vi "ReadData.vi"() -> (7 "Data":T1={"DAQ Config Data"={"Vertical"={"Coupling"=1, "Offset (V)"=-0.5, "Range (V)"=2.0, "Impedance"=50.0}, "Horizontal"={"Offset Time"=0.0, "Sample Time (S)"=22.0, "Sample Points"=1000}, "Trigger\n"={"Lower Level (V)"=-0.02, "Trigger Slope"=1, "Trigger Source"=10}, "Acquisition"={"Trigger Mode"=1, "Initiate Continuously"=0, "Acquire Type"=0, "Acquire Count"=1}, "Channel"=0, "Instrument Handle"=0, "Error"={"status"=FALSE, "code"=0, "source"=""}, "State"=1}, "Acquisition"={"Current"={"Acquiring Now?"=FALSE, "Waveforms Acquired"=0.0, "Start of Acquisition"=timestamp(0 s since 1904-01-01), "Acquisition Name"=""}, "Stop Condition"={"Quota"=3000.0, "Duration (S)"=22, "Stop Condition"=FALSE}, "Config Needed"=FALSE}, "Measurement"={"Waveform"={"t0"=timestamp(0 s since 1904-01-01), "dt"=1.0, "Y"=[]}, "Peak Heights"=[], "Acquisition Time"=timestamp(0 s since 1904-01-01), "File Path"=path "C:/Users/lab-341/Desktop/Reed/Oscilloscope VI/pulses.tdms", "TDMS File Handle"=refnum}, "UI References"={"Acquire"=refnum, "Configure DAQ"=refnum, "Measurement (Ch1)"=refnum, "Update Needed?"=FALSE, "New Run"=refnum, "Signal"=refnum}, "Run Info"={"Active Run?"=FALSE, "Run Notes"="Enter in notes explaining the purpose of the run and any unusual steps taken in the process. This should make it clear why the data was taken. e.g. \"Measuring LXe scintillation light with Teflon\" or \"Measuring dark pulses to determine SPE gain.\" Concise is good but precise is better.", "User Name"="", "Campaign ID#"="", "Run Name"="", "Start Time"=timestamp(0 s since 1904-01-01), "End Time"=timestamp(0 s since 1904-01-01)}, "System Status"={"Bias Voltage"=0.0, "SiPM Temperature"=[], "Slow Control User"="", "LXe"=0.0}, "Acquisition Info"={"Trigger Mode"=FALSE, "Acquisition Mode"=FALSE, "Bias Voltage (V)"=0.0, "Preamplifier"=0, "Shaping Amplifier"=0, "Acquisition Notes"="", "1"=FALSE, "2"=FALSE}} {"Acquisition Info"."Shaping Amplifier" items=["CR-200-100ns", "CR-200-1us"]; "Acquisition Info"."Preamplifier" items=["CR-Z-113-1k", "CR-Z-113-5k", "CR-Z-SiPM"]; "DAQ Config Data"."State" items=["Enable"=1, "Disable"=0]; "DAQ Config Data"."Channel" items=["Input Channel 1", "Input Channel 2", "Input Channel 3", "Input Channel 4"]; "DAQ Config Data"."Acquisition"."Acquire Type" items=["Normal"=0, "Average"=1, "Envelope"=2, "Peak Detect"=3, "High Resolution"=4, "Fast"=5, "Equivalent Time"=16]; "DAQ Config Data"."Acquisition"."Initiate Continuously" items=["Continuously"=1, "Single Capture"=0]; "DAQ Config Data"."Acquisition"."Trigger Mode" items=["Auto", "Normal"]; "DAQ Config Data"."Trigger"."Trigger Source" items=["TTL0", "TTL1", "TTL2", "TTL3", "TTL4", "TTL5", "TTL6", "TTL7", "ECL0", "ECL1", "Input Channel 1", "Input Channel 2", "Input Channel 3", "Input Channel 4", "External Trigger Source", "STAR", "Manual Trigger", "Pattern"]; "DAQ Config Data"."Trigger"."Trigger Slope" items=["Rising Edge", "Falling Edge"]; "DAQ Config Data"."Horizontal"."Sample Time (S)" items=["0.5"=0.5, "0.4"=0.4, "0.25"=0.25, "0.2"=0.2, "0.1"=0.1, "0.05"=0.05, "0.04"=0.04, "0.025"=0.025, "0.02"=0.02, "0.01"=0.01, "0.005"=0.005, "0.004"=0.004, "0.0025"=0.0025, "0.002"=0.002, "0.001"=0.001, "5E-4"=0.0005, "4E-4"=0.0004, "2.5E-4"=0.00025, "2E-4"=0.0002, "1E-4"=0.0001, "5E-5"=5e-05, "4E-5"=4e-05, "2E-5"=2e-05, "5E-6"=5e-06, "1E-6"=1e-06, "5E-7"=5e-07, "1E-7"=1e-07, "5E-8"=5e-08, "1E-8"=1e-08]; "DAQ Config Data"."Vertical"."Impedance" items=["50 Ohm"=50.0, "1 MOhm"=1000000.0]; "DAQ Config Data"."Vertical"."Range (V)" items=["10"=10.0, "5"=5.0, "2"=2.0, "1"=1.0, "0.4"=0.4, "0.2"=0.2, "0.08"=0.08, "0.04"=0.04, "0.02"=0.02, "0.01"=0.01]; "DAQ Config Data"."Vertical"."Coupling" items=["AC", "DC"]})   [LabVIEW 2023]
uses:
  TypeDefs/DataTypes/Data.ctl
  TypeDefs/DataTypes/DAQConfig.ctl
  TypeDefs/DataTypes/Acquisition.ctl
  TypeDefs/DataTypes/Current.ctl
  TypeDefs/DataTypes/StopCondition.ctl
  TypeDefs/DataTypes/Measurement.ctl
  TypeDefs/DataTypes/UIReferences.ctl
  TypeDefs/DataTypes/RunInfo.ctl
  TypeDefs/DataTypes/SystemStatus.ctl
  TypeDefs/Paths/DataPath.ctl
  <vilib>/Utility/xml.llb/Read From XML File(string).vi
panel:
  # "Shaper Gain"
  # "Self"
  # "Fast"
  # "Solicited"
  # "Standard"
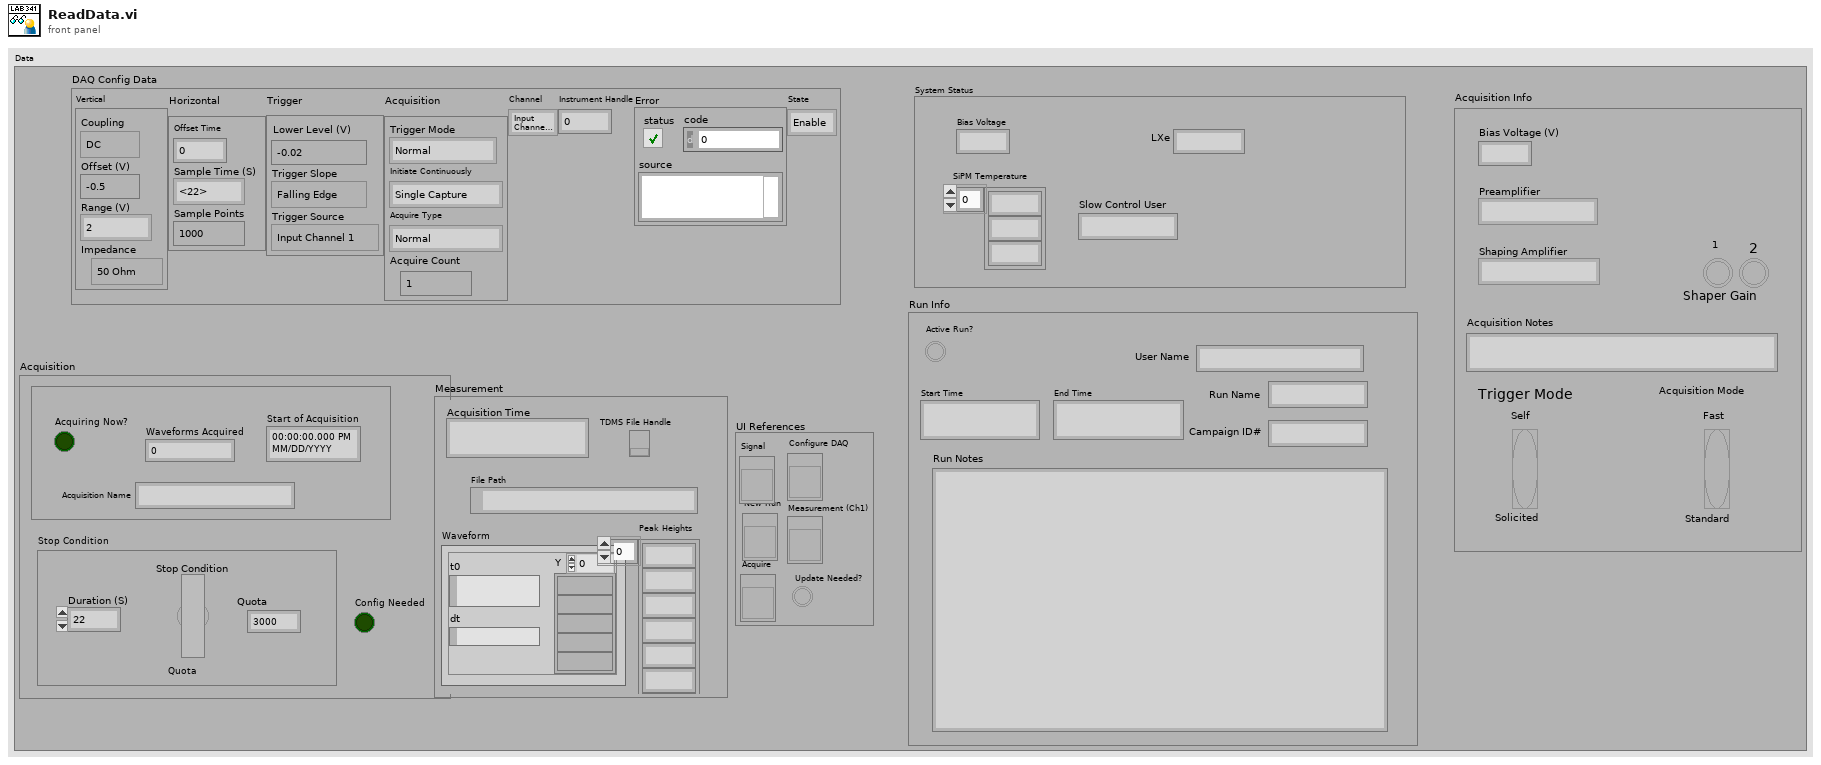
[diagram p1: front panel]
types:
  T1 = typedef "Data.ctl" = cluster{"DAQ Config Data":T2, "Acquisition":T3, "Measurement":T6, "UI References":T7, "Run Info":T8, "System Status":T9, "Acquisition Info":cluster{"Trigger Mode":bool, "Acquisition Mode":bool, "Bias Voltage (V)":dbl, "Preamplifier":u16, "Shaping Amplifier":u16, "Acquisition Notes":string, "1":bool, "2":bool}}
  T2 = typedef "DAQConfig.ctl" = cluster{"Vertical":cluster{"Coupling":i32, "Offset (V)":dbl, "Range (V)":dbl, "Impedance":dbl}, "Horizontal":cluster{"Offset Time":dbl, "Sample Time (S)":dbl, "Sample Points":u32}, "Trigger\n":cluster{"Lower Level (V)":dbl, "Trigger Slope":i32, "Trigger Source":i32}, "Acquisition":cluster{"Trigger Mode":i32, "Initiate Continuously":i32, "Acquire Type":i32, "Acquire Count":i32}, "Channel":i32, "Instrument Handle":i32, "Error":errorcluster, "State":i32}
  T3 = typedef "Acquisition.ctl" = cluster{"Current":T4, "Stop Condition":T5, "Config Needed":bool}
  T4 = typedef "Current.ctl" = cluster{"Acquiring Now?":bool, "Waveforms Acquired":dbl, "Start of Acquisition":timestamp, "Acquisition Name":string}
  T5 = typedef "StopCondition.ctl" = cluster{"Quota":dbl, "Duration (S)":u16, "Stop Condition":bool}
  T6 = typedef "Measurement.ctl" = cluster{"Waveform":waveform(dbl), "Peak Heights":dbl[], "Acquisition Time":timestamp, "File Path":path, "TDMS File Handle":refnum<k34>}
  T7 = typedef "UIReferences.ctl" = cluster{"Acquire":refnum<vi>, "Configure DAQ":refnum<vi>, "Measurement (Ch1)":refnum<vi>, "Update Needed?":bool, "New Run":refnum<vi>, "Signal":refnum<vi>}
  T8 = typedef "RunInfo.ctl" = cluster{"Active Run?":bool, "Run Notes":string, "User Name":string, "Campaign ID#":string, "Run Name":string, "Start Time":timestamp, "End Time":timestamp}
  T9 = typedef "SystemStatus.ctl" = cluster{"Bias Voltage":dbl, "SiPM Temperature":dbl[], "Slow Control User":string, "LXe":dbl}
  T10 = typedef "DataPath.ctl" = path
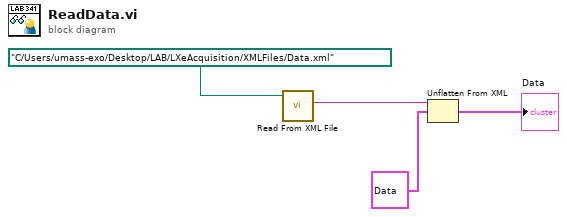
[diagram p0: block diagram]
diagram:
  n1 = call-poly <vilib>:"Read From XML File.vi"("XML File Path"=T10 path "C:/Users/umass-exo/Desktop/LAB/LXeAcquisition/XMLFiles/Data.xml") -> ("XML Elements"=w4:string)  [unwired: 8 in, 2 out]
  n2 = Unflatten From XML(xml string=w4, type=T1 {"DAQ Config Data"={"Vertical"={"Coupling"=1, "Offset (V)"=-0.5, "Range (V)"=2.0, "Impedance"=50.0}, "Horizontal"={"Offset Time"=0.0, "Sample Time (S)"=22.0, "Sample Points"=1000}, "Trigger\n"={"Lower Level (V)"=-0.02, "Trigger Slope"=1, "Trigger Source"=10}, "Acquisition"={"Trigger Mode"=1, "Initiate Continuously"=0, "Acquire Type"=0, "Acquire Count"=0}, "Channel"=0, "Instrument Handle"=0, "Error"={"status"=FALSE, "code"=0, "source"=""}, "State"=1}, "Acquisition"={"Current"={"Acquiring Now?"=FALSE, "Waveforms Acquired"=0.0, "Start of Acquisition"=timestamp(0 s since 1904-01-01), "Acquisition Name"=""}, "Stop Condition"={"Quota"=3000.0, "Duration (S)"=22, "Stop Condition"=FALSE}, "Config Needed"=FALSE}, "Measurement"={"Waveform"={"t0"=timestamp(0 s since 1904-01-01), "dt"=1.0, "Y"=[]}, "Peak Heights"=[], "Acquisition Time"=timestamp(0 s since 1904-01-01), "File Path"=path "", "TDMS File Handle"=refnum}, "UI References"={"Acquire"=refnum, "Configure DAQ"=refnum, "Measurement (Ch1)"=refnum, "Update Needed?"=FALSE, "New Run"=refnum, "Signal"=refnum}, "Run Info"={"Active Run?"=FALSE, "Run Notes"="Enter in notes explaining the purpose of the run and any unusual steps taken in the process. This should make it clear why the data was taken. e.g. \"Measuring LXe scintillation light with Teflon\" or \"Measuring dark pulses to determine SPE gain.\" Concise is good but precise is better.", "User Name"="", "Campaign ID#"="", "Run Name"="", "Start Time"=timestamp(0 s since 1904-01-01), "End Time"=timestamp(0 s since 1904-01-01)}, "System Status"={"Bias Voltage"=0.0, "SiPM Temperature"=[], "Slow Control User"="", "LXe"=0.0}, "Acquisition Info"={"Trigger Mode"=FALSE, "Acquisition Mode"=FALSE, "Bias Voltage (V)"=0.0, "Preamplifier"=0, "Shaping Amplifier"=0, "Acquisition Notes"="", "1"=FALSE, "2"=FALSE}} ("Data")) -> (value=→"Data":T1)  [unwired: 1 in, 1 out]
